vi "Andor Test.vi"() -> ()   [LabVIEW 2018, in "Andor Camera.lvlib"]
uses:
  Andor Camera.lvlib
  <userlib>/atmcd64d.llb/AcquisitionMode_mode typedef.ctl
  <userlib>/atmcd64d.llb/ReadMode_mode typedef.ctl
  <userlib>/atmcd64d.llb/TriggerMode_mode typedef.ctl
  <userlib>/atmcd64d.llb/HSSpeed_type typedef.ctl
  <userlib>/atmcd64d.llb/Shutter_type typedef.ctl
  <userlib>/atmcd64d.llb/Shutter_mode typedef.ctl
panel:
  out "VS speed":sgl format="%.2f"
  out "Initialize":u32
  out "Acquiring":bool
  out "Intensity Graph":i32[][](graph)
  out "SetTriggerMode":u32
  out "SetVSSpeed":u32
  out "SetHSSpeed":u32
  out "GetMostRecentImage":u32
  out "Image Array":i32[](array[numeric]) caption="Array"
  in  "stop":bool
  out "Shutdown":u32
  out "GetDetector":u32
  out "Y Pixels":i32
  out "Total number of pixels":i32
  out "SetImage":u32
  out "X Pixels":i32
  out "SetExposureTime":u32
  out "SetReadMode":u32
  out "SetAcquisition Mode":u32
  out "Start Acquisition":u32
  in  "Exposure Time (secs)":sgl=0.1 format="%.2f"
  # "INPUT"
  # "Return Values"
  # "Numerical data"
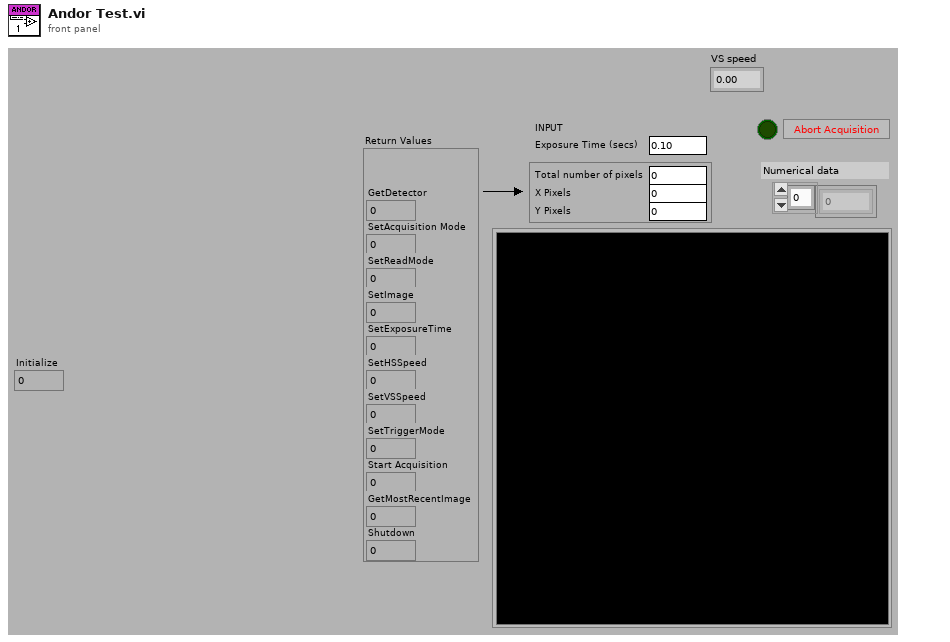
[diagram p1: front panel]
types:
  T1 = typedef "Shutter_mode typedef.ctl" = enum16{"Auto", "Open", "Close", "N/A (3)", "Open FVB Series", "Open Any Series"}
  T2 = typedef "Shutter_type typedef.ctl" = enum16{"TTL Low", "TTL High"}
  T3 = typedef "HSSpeed_type typedef.ctl" = enum16{"EM Amp", "Conventional Amp"}
  T4 = typedef "TriggerMode_mode typedef.ctl" = enum16{"Internal", "External", "N/A (2)", "N/A (3)", "N/A (4)", "N/A (5)", "External Start", "External Exposure (Bulb)", "N/A (8)", "External FVB EM", "Software", "N/A (11)", "External Charge Shifting"}
  T5 = typedef "ReadMode_mode typedef.ctl" = enum16{"Full Vertical Binning", "Multi-Track", "Random-Track", "Single-Track", "Image"}
  T6 = typedef "AcquisitionMode_mode typedef.ctl" = enum16{"Reserved (0)", "Single Scan", "Accumulate", "Kinetics", "Fast Kinetics", "Run Till Abort", "Reserved (6)", "Reserved (7)", "Reserved (8)", "Time Delayed Integration"}
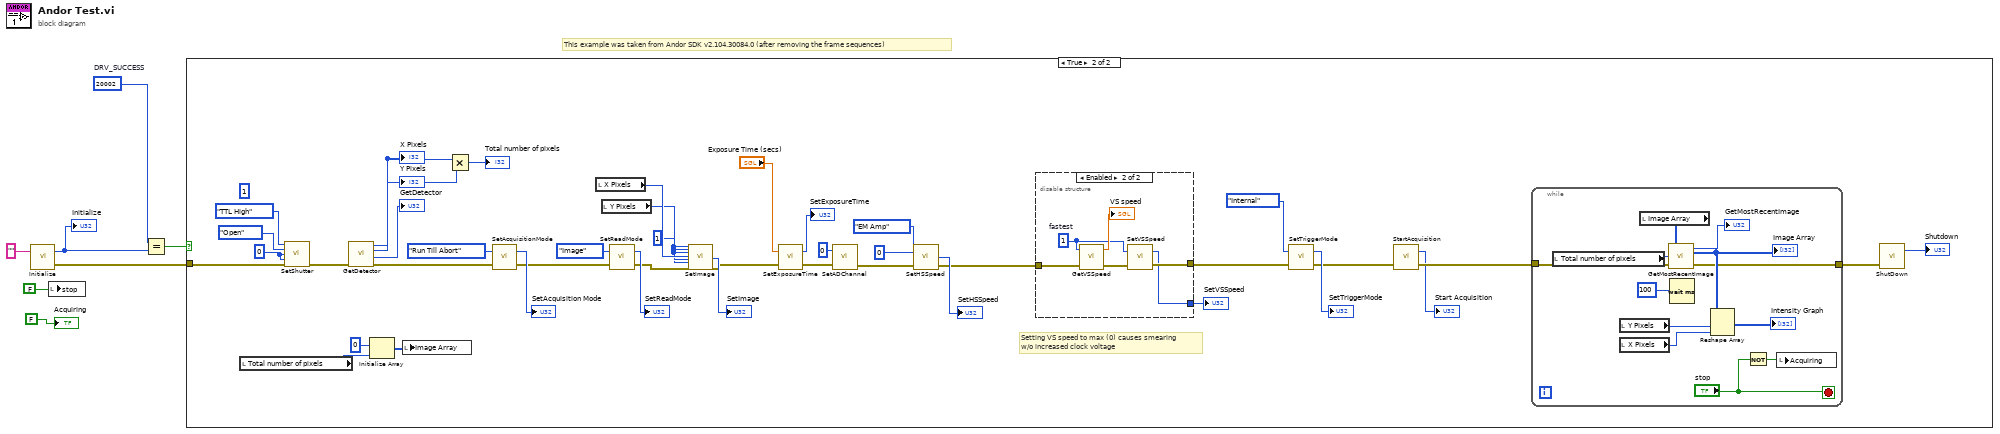
[diagram p0: block diagram]
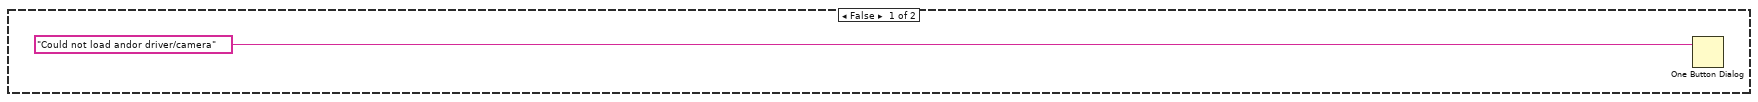
[diagram p2: hidden frame]
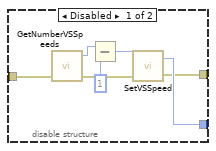
[diagram p3: hidden frame]
diagram:
  w4 = 20002  # DRV_SUCCESS
  # "This example was taken from Andor SDK v2.104.30084.0 (after removing the frame sequences)"
  n1 = call <userlib>:"Initialize.vi"("directory (\"\")"="") -> ("error out"=w2:errorcluster, "DLL error code"=w6:u32)  [unwired: 1 in]
  "Initialize" <- w6
  n2 = local write "stop"(FALSE) -> ()
  n3 = Equal?(x=w4, y=w6) -> (x = y?=w5:bool)
  n4 = case shown="True" w5 {
    tunnel: w2 -> [_ w49]
    frame False {
      n5 = One Button Dialog(message="Could not load andor driver/camera") -> ()  [unwired: 1 in, 1 out]
    }
    frame True {
      w40 = 1
      (unwired) 1
      w9 = 0
      # "Setting VS speed to max (0) causes smearing\nw/o increased clock voltage"
      n6 = local read "Total number of pixels"() -> (w29:i32)
      n7 = call <userlib>:"SetShutter.vi"("type"=Shutter_type_typedef."TTL High", "mode"=Shutter_mode_typedef."Open", "closingtime"=w9, "openingtime"=w9, "error in (no error)"=w49) -> ("error out"=w26:errorcluster)  [unwired: 9 in, 1 out]
      n8 = call <userlib>:"GetDetector.vi"("error in (no error)"=w26) -> ("error out"=w25:errorcluster, "DLL error code"=→"GetDetector":u32, "ypixels"=w46:i32, "xpixels"=w45:i32)  [unwired: 3 in]
      "X Pixels" <- w45
      "Y Pixels" <- w46
      n9 = Initialize Array(0, w29) -> (w28:i32[])
      n10 = local write "Image Array"(w28) -> ()
      n11 = Multiply(x=w45, y=w46) -> (x*y=→"Total number of pixels":i32)
      n12 = call <userlib>:"SetAcquisitionMode.vi"("error in (no error)"=w25, "mode"=AcquisitionMode_mode_typedef."Run Till Abort") -> ("error out"=w24:errorcluster, "DLL error code"=→"SetAcquisition Mode":u32)
      n13 = local read "X Pixels"() -> (w41:i32)
      n14 = local read "Y Pixels"() -> (w39:i32)
      n15 = call <userlib>:"SetReadMode.vi"("error in (no error)"=w24, "mode"=ReadMode_mode_typedef."Image") -> ("error out"=w23:errorcluster, "DLL error code"=→"SetReadMode":u32)
      n16 = call <userlib>:"SetImage.vi"("hbin"=w40, "vbin"=w40, "hstart"=w40, "hend"=w41, "vstart"=w40, "vend"=w39, "error in (no error)"=w23) -> ("DLL error code"=→"SetImage":u32, "error out"=w22:errorcluster)  [unwired: 19 in]
      n17 = call <userlib>:"SetExposureTime.vi"("error in (no error)"=w22, "time"="Exposure Time (secs)") -> ("error out"=w21:errorcluster, "DLL error code"=→"SetExposureTime":u32)
      n18 = call <userlib>:"SetADChannel.vi"("error in (no error)"=w21, "channel"=0) -> ("error out"=w20:errorcluster)  [unwired: 1 out]
      n19 = call <userlib>:"SetHSSpeed.vi"("error in (no error)"=w20, "index"=0 ("input param"), "type"=HSSpeed_type_typedef."EM Amp") -> ("error out"=w19:errorcluster, "DLL error code"=→"SetHSSpeed":u32)  [unwired: 1 in]
      n20 = disable-structure shown="Enabled" {
        disable-tunnel: [w57 w58] -> w32
        disable-tunnel: w19 -> [w53 w60]
        disable-tunnel: [w51 w59] -> w18
        frame Disabled {
          n21 = call <userlib>:"GetNumberVSSpeeds.vi"("error in (no error)"=w53) -> ("error out"=w52:errorcluster, "number"=w56:i32)  [unwired: 2 in, 1 out]
          n22 = Subtract(x=w56, y=1) -> (x-y=w54:i32)
          n23 = call <userlib>:"SetVSSpeed.vi"("error in (no error)"=w52, "index"=w54) -> ("error out"=w51:errorcluster, "DLL error code"=w57:u32)
        }
        frame Enabled {
          w61 = 1  # fastest
          n24 = call <userlib>:"GetVSSpeed.vi"("error in (no error)"=w60, "index"=w61) -> ("error out"=w62:errorcluster, "speed"=→"VS speed":sgl)  [unwired: 1 in, 1 out]
          n25 = call <userlib>:"SetVSSpeed.vi"("error in (no error)"=w62, "index"=w61) -> ("error out"=w59:errorcluster, "DLL error code"=w58:u32)
        }
      }
      "SetVSSpeed" <- w32
      n26 = call <userlib>:"SetTriggerMode.vi"("error in (no error)"=w18, "mode"=TriggerMode_mode_typedef."Internal") -> ("error out"=w17:errorcluster, "DLL error code"=→"SetTriggerMode":u32)
      n27 = call <userlib>:"StartAcquisition.vi"("error in (no error)"=w17) -> ("error out"=w50:errorcluster, "DLL error code"=→"Start Acquisition":u32)  [unwired: 1 in]
      n28 = while {
        tunnel: w50 -> [w69]
        tunnel: [w68] -> w48
        stop <- "stop" stop-if-true
        n29 = local read "Total number of pixels"() -> (w66:i32)
        n30 = local read "Y Pixels"() -> (w73:i32)
        n31 = local read "X Pixels"() -> (w72:i32)
        n32 = local read "Image Array"() -> (w65:i32[])
        n33 = call <userlib>:"GetMostRecentImage.vi"("error in (no error)"=w69, "size"=w66, "array"=w65) -> ("error out"=w68:errorcluster, "array"=w75:i32[], "DLL error code"=→"GetMostRecentImage":u32)
        "Image Array" <- w75
        n34 = Wait (ms)(milliseconds to wait=100) -> ()  [unwired: 1 out]
        n35 = Reshape Array(w75, w73, w72) -> (→"Intensity Graph":i32[][])
        n36 = Not(x="stop") -> (.not. x?=w71:bool)
        n37 = local write "Acquiring"(w71) -> ()
      }
      n38 = call <userlib>:"ShutDown.vi"("error in (no error)"=w48) -> ("DLL error code"=→"Shutdown":u32)  [unwired: 1 in, 1 out]
    }
  }
  "Acquiring" <- FALSE
